vi "HIOKI PW3390 Acquisition Efficiency.vi"() -> ()   [LabVIEW 2009]
doc: "Outputs the results of Efficiency/Loss calculation in 100ms cycle."
uses:
  <instrlib>/PW3390/Common/_Initialize/HIOKI PW3390 Initialize LAN.vi
  <instrlib>/PW3390/Common/_Initialize/HIOKI PW3390 Initialize RS-232C.vi
panel:
  in  "Item":T1(array[cluster])=[{"Item"=enum."EFFI", "Ch(0:Ch1)"=enum."1"}, {"Item"=enum."EFFI", "Ch(0:Ch1)"=enum."2"}, {"Item"=enum."EFFI", "Ch(0:Ch1)"=enum."3"}, {"Item"=enum."LOSS", "Ch(0:Ch1)"=enum."1"}, {"Item"=enum."LOSS", "Ch(0:Ch1)"=enum."2"}, {"Item"=enum."LOSS", "Ch(0:Ch1)"=enum."3"}]
  in  "Pout (0: P1)":T2(array[ring])=[enum."P1", enum."P1", enum."P1"]
  in  "Pin (0: P1)":T2(array[ring])=[enum."P1", enum."P1", enum."P1"]
  out "Data out":dbl[](array[numeric])
  out "error out":errorcluster
  in  "Stop":bool
  in  "Communication Interface":enum16{"LAN", "RS-232C"}(ring)
  in  "COM Port":refnum<visa-resource-name>="COM1"
  in  "baud rate (38400bps)":u32=38400
  in  "IP Address":string="192.168.1.1"
  # "Note:\n Please set configuration before starting the program.\nChanging configuration during running the program is invalid."
  # "Pin1           Pin2           Pin3"
  # "Pout1         Pout2         Pout3"
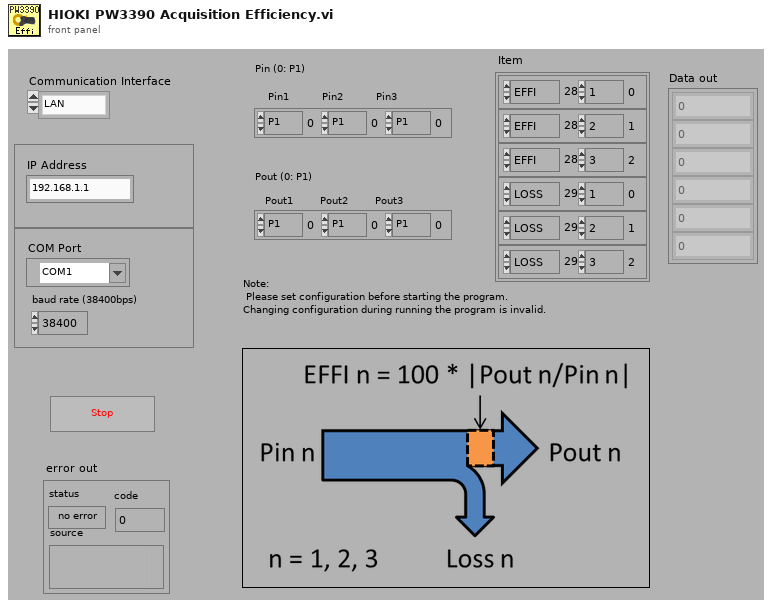
[diagram p1: front panel]
types:
  T1 = cluster{"Item":enum16{"Urms", "Umn", "Uac", "Udc", "Ufnd", "Upk+", "Upk-", "Uthd", "Urf", "Uunb", "Irms", "Imn", "Iac", "Idc", "Ifnd", "Ipk+", "Ipk-", "Ithd", "Irf", "Iunb", "P", "S", "Q", "PF", "DEG U", "DEG I", "DEG P", "f", "EFFI", "LOSS", "IH+", "IH-", "IH", "WP+", "WP-", "WP", "CH A", "CH B", "Pm", "Slip", "Laptime", "Laptime(ms)"}, "Ch(0:Ch1)":enum16{"1", "2", "3", "4", "12", "34", "123"}}[]
  T2 = enum16{"P1", "P2", "P3", "P4", "P12", "P34", "P123", "Pm"}[]
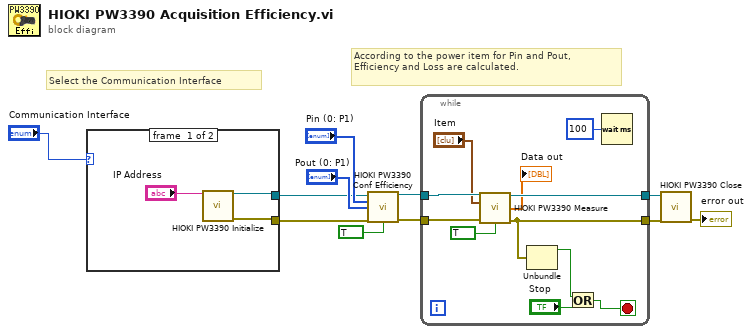
[diagram p0: block diagram]
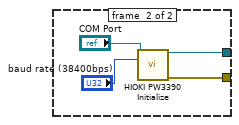
[diagram p2: hidden frame]
diagram:
  # "According to the power item for Pin and Pout,\nEfficiency and Loss are calculated."
  # "Select the Communication Interface"
  n1 = case shown="\"LAN\", デフォルト" "Communication Interface" {
    tunnel: [w13 w18] -> w5
    tunnel: [w12 w17] -> w4
    frame #0 {
      n2 = call-poly <instrlib>:"HIOKI PW3390 Initialize.vi"("IP Address"="IP Address") -> ("VISA Resource out"=w13:refnum<visa-resource-name>, "error out"=w12:errorcluster)  [unwired: 12 in, 1 out]
    }
    frame #1 {
      n3 = call-poly <instrlib>:"HIOKI PW3390 Initialize.vi"("COM Port"="COM Port", "baud rate (38400bps)"="baud rate (38400bps)") -> ("VISA Resource out"=w18:refnum<visa-resource-name>, "error out"=w17:errorcluster)  [unwired: 11 in, 1 out]
    }
  }
  n4 = call <instrlib>:"HIOKI PW3390 Conf Efficiency.vi"("VISA Resource"=w5, "Pin (0: P1)"="Pin (0: P1)", "Pout (0: P1)"="Pout (0: P1)", "error in (no error)"=w4, "Error Out (F: Off)"=TRUE) -> ("VISA Resource out"=w3:refnum<visa-resource-name>, "error out"=w2:errorcluster)  [unwired: 7 in, 2 out]
  n5 = while {
    tunnel: w3 -> [w22]
    tunnel: w2 -> [w21]
    tunnel: [w25] -> w10
    tunnel: [w24] -> w9
    stop <- w27 stop-if-true
    n6 = call <instrlib>:"HIOKI PW3390 Measure.vi"("VISA Resource"=w22, "Item"="Item", "error in (no error)"=w21, "Error Out (F: Off)"=TRUE) -> ("VISA Resource out"=w25:refnum<visa-resource-name>, "Data out"=→"Data out":dbl[], "error out"=w24:errorcluster)  [unwired: 6 in, 3 out]
    n7 = Unbundle(w24) -> ("status"=w28:bool)  [unwired: 2 out]
    n8 = Or(x=w28, y="Stop") -> (x .or. y?=w27:bool)
    n9 = Wait (ms)(milliseconds to wait=u32 100) -> ()  [unwired: 1 out]
  }
  n10 = call <instrlib>:"HIOKI PW3390 Close.vi"("VISA Resource"=w10, "error in (no error)"=w9) -> ("error out"=→"error out":errorcluster)  [unwired: 13 in]
